vi "NotifyObserver.vi"(8 "error in":errorcluster, 9 "ObservableDataValue":variant[](array[variant]), 10 "ObservableDataName":string[](array[string]), 11 "IstanceName":string) -> (0 "error out":errorcluster)   [LabVIEW 2025, in "ObserverClass.lvlib"]
doc: "Send Notification to all the Observer"
uses:
  ObserverClass.lvlib
  ObserverClass/Controls/observerControl.ctl
  ObserverClass/ObserverClass.lvclass
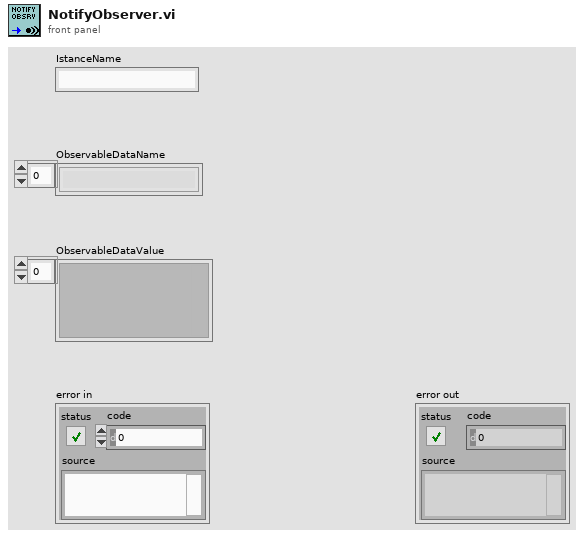
[diagram p1: front panel]
types:
  T1 = enum16{"Get", "Set", "Init", "Remove", "Destroy"}
  T2 = typedef "ObserverClass.lvlib/ObserverClass.lvclass/observerControl.ctl" = cluster{"ObservableName":string, "ObservableValue":variant, "SenderName":string}
  T3 = map{string, cluster{"ObserverEvent":refnum<user-event>, "ObserverNr":u64, "Value":variant}}
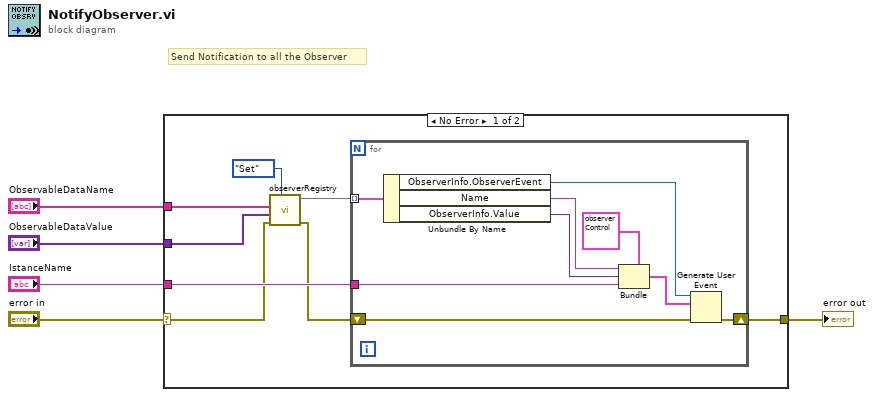
[diagram p0: block diagram]
diagram:
  # "Send Notification to all the Observer"
  n1 = case shown="No Error" "error in" {
    selector: "error in" -> [w7 w23]
    tunnel: "ObservableDataName" -> [w12 _]
    tunnel: "ObservableDataValue" -> [w10 _]
    tunnel: "IstanceName" -> [w9 _]
    tunnel: [w8 w23] -> w5
    frame No Error {
      n2 = call "observerRegistry.vi"("Action"=T1."Set", "error in"=w7, "ObservableValue"=w10, "ObservableName"=w12) -> ("error out"=w6:errorcluster, "Observable out"=w11:T3)  [unwired: 5 in, 1 out]
      n3 = for {
        tunnel: w11 -> [w22] mode=indexing
        tunnel: w9 -> [w17]
        shift-right: [w14] -> w8
        shift-left: w6 -> [w15]
        n4 = Unbundle By Name(w22) -> ("ObserverInfo.ObserverEvent"=w21:refnum<user-event>, "Name"=w18:string, "ObserverInfo.Value"=w16:variant)
        n5 = Bundle(cluster=T2 {"ObservableName"="", "ObservableValue"=variant, "SenderName"=""} ("event data"), "ObservableName"=w18, "ObservableValue"=w16, "SenderName"=w17) -> (w20:T2)
        n6 = Generate User Event(user event=w21, event data cluster=w20, error in=w15) -> (error out=w14:errorcluster)  [unwired: 1 in, 1 out]
      }
    }
    frame Error {
    }
  }
  "error out" <- w5
